vi "MT Generate MSK Synchronization Parameters (bit array).vi"(0 "MSK system parameters":T1={"differential encoding enable"=enum."disable", "samples per symbol (16)"=16}, 1 "symbol rate (Hz)":dbl format="%.2f", 5 "sync bits":i8[](array[numeric]), 11 "error in (no error)":errorcluster, 12 "expected sync location (symbols)":i32=-1, 13 "sync location uncertainty (symbols)":i32=10, 14 "sync indent (symbols)":i32) -> (4 "MSK synchronization parameters":T2 {"sync sequence" format="%.2f"}, 15 "error out":errorcluster)   [LabVIEW 2020, in "niDMT.lvlib"]
doc: "This polymorphic instance generates synchronization parameters for MSK demodulation using a synchronization sequence directly represented by the <B>sync bits</B> input array."
uses:
  <vilib>/addons/Modulation/niDMT.lvlib
  <vilib>/addons/Modulation/niAMT.lvlib
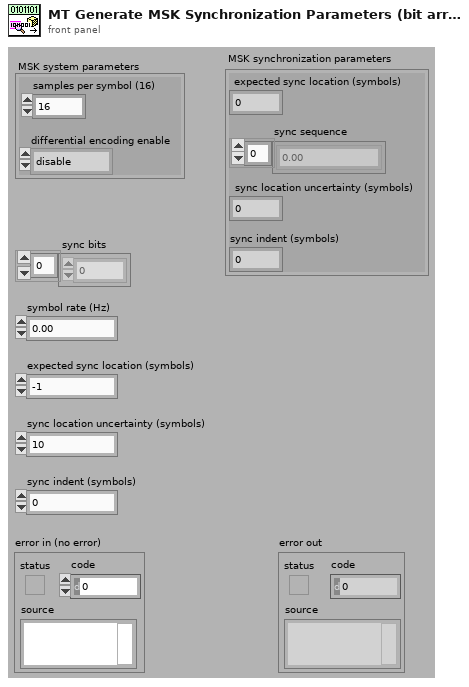
[diagram p1: front panel]
types:
  T1 = cluster{"differential encoding enable":enum16{"disable", "enable"}, "samples per symbol (16)":i32}
  T2 = cluster{"expected sync location (symbols)":i32, "sync sequence":cdb[], "sync location uncertainty (symbols)":i32, "sync indent (symbols)":i32}
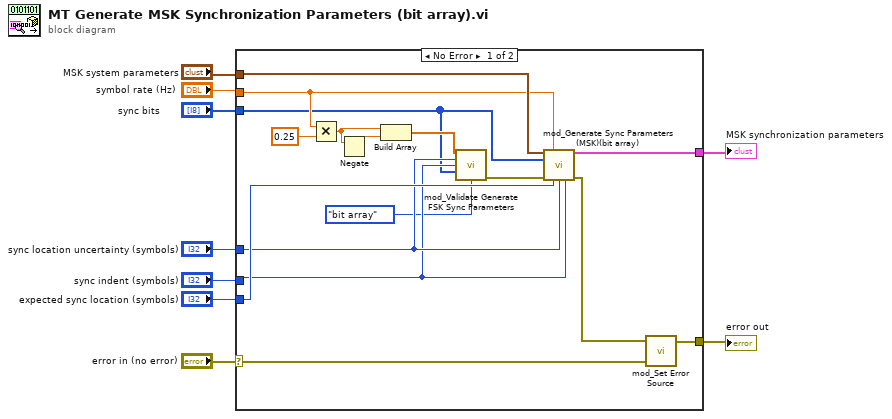
[diagram p0: block diagram]
diagram:
  n1 = case shown="No Error" "error in (no error)" {
    selector: "error in (no error)" -> [w22 w26]
    tunnel: "expected sync location (symbols)" -> [w20 _]
    tunnel: "sync location uncertainty (symbols)" -> [w13 _]
    tunnel: "sync indent (symbols)" -> [w12 _]
    tunnel: "sync bits" -> [w11 _]
    tunnel: [w25 w26] -> w4
    tunnel: "MSK system parameters" -> [w21 _]
    tunnel: "symbol rate (Hz)" -> [w18 _]
    tunnel: [w24 _] -> w1
    frame No Error {
      n2 = Multiply(x=w18, y=0.25) -> (x*y=w16:dbl)
      n3 = Negate(x=w16) -> (-x=w15:dbl)
      n4 = Build Array(w16, w15) -> (w14:dbl[])
      n5 = call <vilib>:"mod_Validate Generate FSK Sync Parameters.vi"("symbol map"=w14, "sync location uncertainty (symbols)"=w13, "sync indent (symbols)"=w12, "sync bits"=w11, "sync bits specification"=enum16{"bit array", "number array", "number"}."bit array") -> ("error out"=w19:errorcluster)  [unwired: 2 in, 8 out]
      n6 = call <vilib>:"mod_Generate Sync Parameters (MSK)(bit array).vi"("MSK system parameters"=w21, "symbol rate (Hz)"=w18, "sync bits"=w11, "error in (no error)"=w19, "expected sync location (symbols)"=w20, "sync location uncertainty (symbols)"=w13, "sync indent (symbols)"=w12) -> ("MSK synchronization parameters"=w24:T2, "error out"=w23:errorcluster)  [unwired: 7 out]
      n7 = call <vilib>:"mod_Set Error Source.vi"("initial error in (no error)"=w22, "final error in (no error)"=w23) -> ("error out"=w25:errorcluster)  [unwired: 3 out]
    }
    frame Error {
    }
  }
  "MSK synchronization parameters" <- w1
  "error out" <- w4
